vi "Parse CfgTable(with DataName).vi"(7 "Cluster Configuration Typedef":variant, 8 "error in (no error)":errorcluster, 11 "CfgTable Row":string[](array[string])) -> (0 "error out":errorcluster, 1 "Elements":i32, 3 "Cluster Configuration Out":variant)   [LabVIEW 2017, in "ClusterCfgTable.lvlib"]
doc: "NEVSTOP-Programming-Palette 2021.12.23.1\nNEVSTOP - NEVSTOP\nCopyright (c) 2021, NEVSTOP"
uses:
  ClusterCfgTable.lvlib
  <userlib>/_OpenG.lib/string/string.llb/Trim Whitespace (String)__ogtk.vi
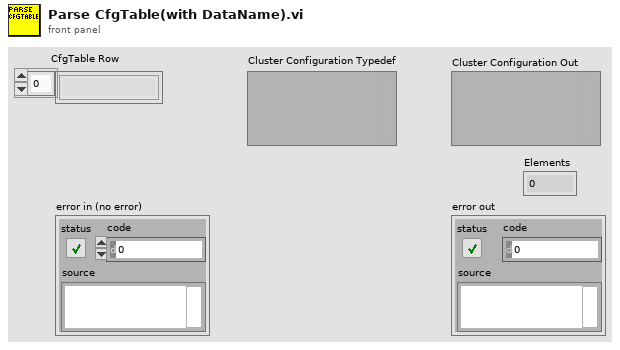
[diagram p1: front panel]
types:
  T1 = typedef "Type Descriptor Enumeration__ogtk.ctl" = enum8{"<Null>", "I8", "I16", "I32", "I64", "U8", "U16", "U32", "U64", "SGL", "DBL", "EXT", "CSG", "CDB", "CXT", "0x0F", "0x10", "0x11", "0x12", "0x13", "0x14", "Enum U8", "Enum U16", "Enum U32", "Enum U64", "SGL PQ", "DBL PQ", "EXT PQ", "CSG PQ", "CDB PQ", "CXT PQ", "0x1F", "0x20", "Boolean", "0x22", "0x23", "0x24", "0x25", "0x26", "0x27", "0x28", "0x29", "0x2A", "0x2B", "0x2C", "0x2D", "0x2E", "0x2F", "String", "0x31", "Path", "Pict", "0x34", "0x35", "0x36", "DAQ", "0x38", "0x39", "0x3A", "0x3B", "0x3C", "0x3D", "0x3E", "0x3F", "Array", "0x41", "0x42", "0x43", "0x44", "0x45", "0x46", "0x47", "0x48", "0x49", "0x4A", "0x4B", "0x4C", "0x4D", "0x4E", "0x4F", "Cluster", "0x51", "0x52", "Variant", "Waveform", "0x55", "0x56", "0x57", "0x58", "0x59", "0x5A", "0x5B", "0x5C", "0x5D", "0x5E", "0x5F", "0x60", "0x61", "0x62", "0x63", "0x64", "0x65", "0x66", "0x67", "0x68", "0x69", "0x6A", "0x6B", "0x6C", "0x6D", "0x6E", "0x6F", "Refnum"}
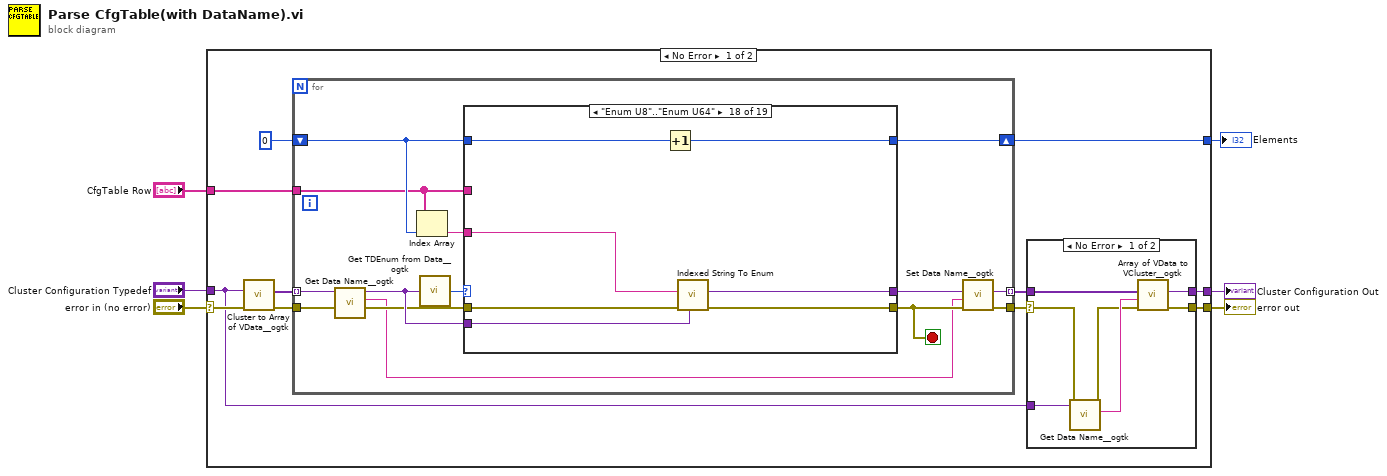
[diagram p0: block diagram]
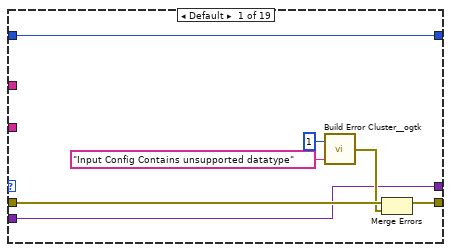
[diagram p3: hidden frame]
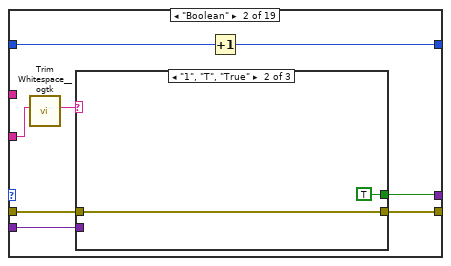
[diagram p4: hidden frame]
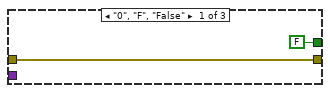
[diagram p5: hidden frame]
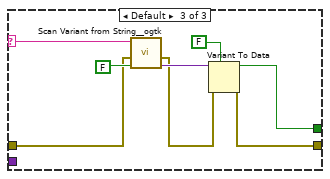
[diagram p6: hidden frame]
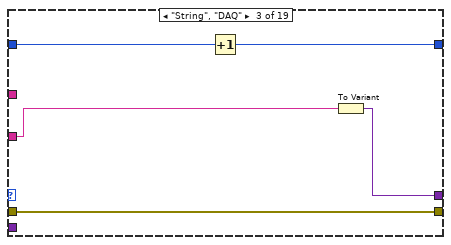
[diagram p7: hidden frame]
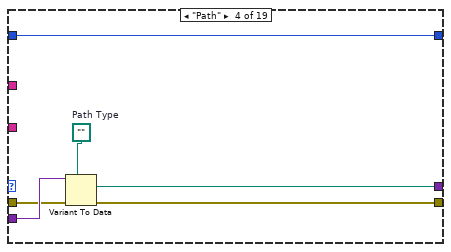
[diagram p8: hidden frame]
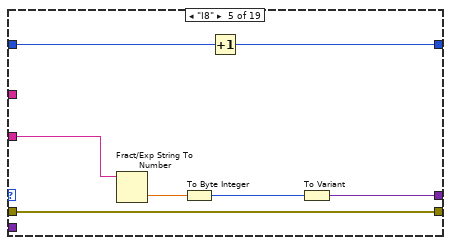
[diagram p9: hidden frame]
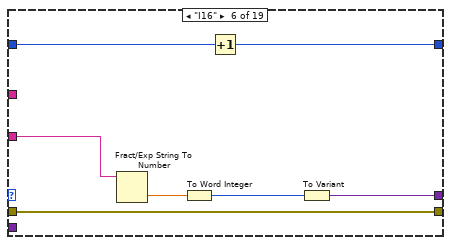
[diagram p10: hidden frame]
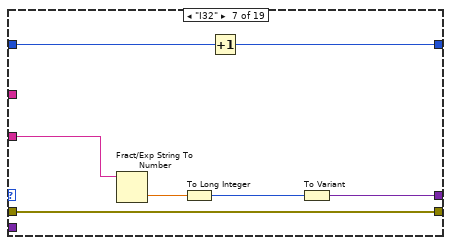
[diagram p11: hidden frame]
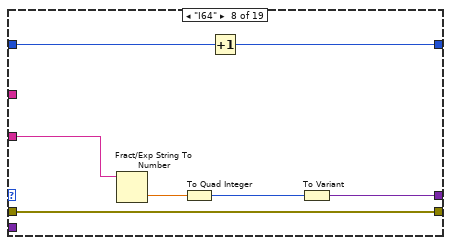
[diagram p12: hidden frame]
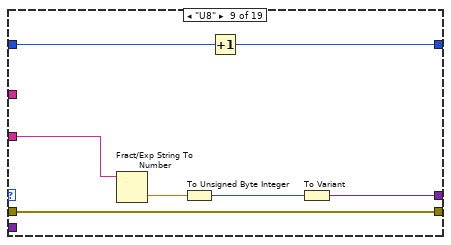
[diagram p13: hidden frame]
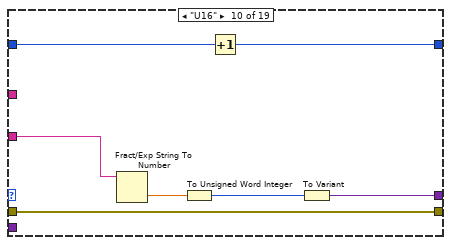
[diagram p14: hidden frame]
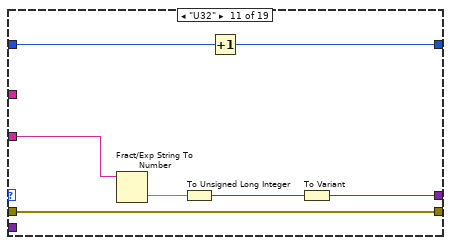
[diagram p15: hidden frame]
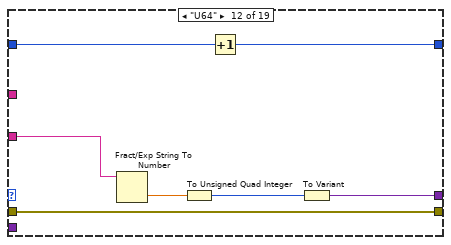
[diagram p16: hidden frame]
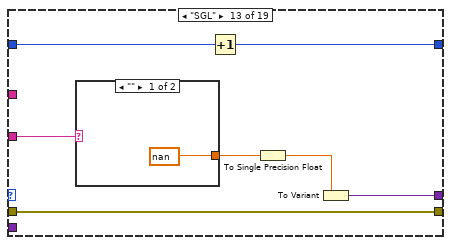
[diagram p17: hidden frame]
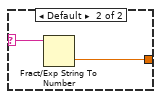
[diagram p18: hidden frame]
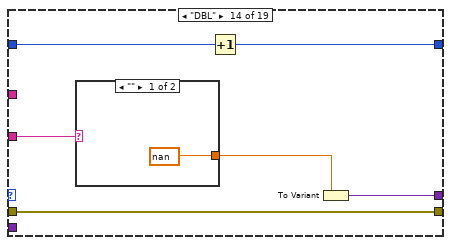
[diagram p19: hidden frame]
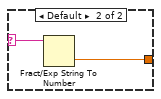
[diagram p20: hidden frame]
diagram:
  n1 = case shown="No Error" "error in (no error)" {
    selector: "error in (no error)" -> [w12 w201]
    tunnel: "CfgTable Row" -> [w17 _]
    tunnel: [w16 w200] -> w5
    tunnel: [w15 w201] -> w4
    tunnel: "Cluster Configuration Typedef" -> [w8 w200]
    tunnel: [w7 _] -> w1
    frame No Error {
      n2 = call <userlib>:"Cluster to Array of VData__ogtk.vi"("error in (no error)"=w12, "Cluster"=w8) -> ("error out"=w13:errorcluster, "Array of VData"=w10:variant[])  [unwired: 8 in]
      n3 = for {
        tunnel: w17 -> [w34]
        tunnel: w10 -> [w37] mode=indexing
        tunnel: [w30] -> w11 mode=indexing
        tunnel: w13 -> [w32]
        tunnel: [w28] -> w14
        shift-right: [w36] -> w7
        shift-left: 0 -> [w35]
        stop <- w29 stop-if-true
        n4 = call <userlib>:"Get Data Name__ogtk.vi"("error in (no error)"=w32, "Data"=w37) -> ("error out"=w31:errorcluster, "Data Name"=w27:string, "Data dup"=w33:variant)  [unwired: 7 in]
        n5 = Index Array(array=w34, index=w35) -> (element=w39:string)
        n6 = call <userlib>:"Get TDEnum from Data__ogtk.vi"("Data"=w33) -> ("Type Descriptor Enumeration"=w40:T1)  [unwired: 4 in]
        n7 = case shown="\"Enum U8\"..\"Enum U64\"" w40 {
          tunnel: w39 -> [_ w55 w72 _ w80 w87 w94 w101 w108 w115 w122 w129 w140 w149 w159 w169 w179 w190 _]
          tunnel: [w42 w53 w71 w74 w85 w92 w99 w106 w113 w120 w127 w134 w141 w150 w160 w170 w180 w189 w195] -> w38
          tunnel: w33 -> [w42 w54 _ w76 _ _ _ _ _ _ _ _ _ _ _ _ _ w188 w196]
          tunnel: w31 -> [w47 w51 w70 w75 w83 w90 w97 w104 w111 w118 w125 w132 w139 w148 w158 w168 w178 w187 w199]
          tunnel: [w46 w50 w70 w73 w83 w90 w97 w104 w111 w118 w125 w132 w139 w148 w158 w168 w178 w186 w192] -> w29
          tunnel: w35 -> [w41 w49 w69 w78 w82 w89 w96 w103 w110 w117 w124 w131 w138 w147 w157 w167 w177 w185 w194]
          tunnel: [w41 w48 w68 w78 w81 w88 w95 w102 w109 w116 w123 w130 w137 w146 w156 w166 w176 w184 w193] -> w36
          tunnel: w34 -> [_ _ _ _ _ _ _ _ _ _ _ _ _ _ _ _ _ _ w198]
          frame Default {
            n8 = call <userlib>:"Build Error Cluster__ogtk.vi"("String to Prepend to source (\"\")"="Input Config Contains unsupported datatype" ("String to Prepend to source (\"\")"), "code"=1) -> ("error out"=w45:errorcluster)
            n9 = Merge Errors(w47, w45) -> (w46:errorcluster)
          }
          frame "Boolean" {
            n10 = call-poly <userlib>:"Trim Whitespace__ogtk.vi"("String in"=w55) -> ("String out"=w52:string)  [unwired: 6 in]
            n11 = case shown="\"1\", \"T\", \"True\"" w52 {
              selector: w52 -> [_ _ w67]
              tunnel: w54 -> [_ _ _]
              tunnel: [FALSE TRUE w64] -> w53
              tunnel: w51 -> [w56 w58 w62]
              tunnel: [w56 w58 w60] -> w50
              frame "0", "F", "False" {
              }
              frame "1", "T", "True" {
              }
              frame Default {
                n12 = call <userlib>:"Scan Variant from String__ogtk.vi"("Default Value"=FALSE, "error in (no error)"=w62, "Input String"=w67) -> ("Output"=w66:variant, "error out"=w61:errorcluster)  [unwired: 5 in, 2 out]
                n13 = Variant To Data(error in=w61, type=FALSE, Variant=w66) -> (data=w64:bool, error out=w60:errorcluster)
              }
            }
            n14 = Increment(x=w49) -> (x+1=w48:i32)
          }
          frame "String", "DAQ" {
            n15 = Increment(x=w69) -> (x+1=w68:i32)
            n16 = To Variant(anything=w72) -> (Variant=w71:variant)
          }
          frame "Path" {
            w77 = path ""  # Path Type
            n17 = Variant To Data(error in=w75, type=w77, Variant=w76) -> (data=w74:path, error out=w73:errorcluster)
          }
          frame "I8" {
            n18 = Fract/Exp String To Number(string=w80) -> (number=w84:dbl)  [unwired: 3 in, 1 out]
            n19 = To Byte Integer(number=w84) -> (8bit integer=w79:i8)
            n20 = Increment(x=w82) -> (x+1=w81:i32)
            n21 = To Variant(anything=w79) -> (Variant=w85:variant)
          }
          frame "I16" {
            n22 = Fract/Exp String To Number(string=w87) -> (number=w91:dbl)  [unwired: 3 in, 1 out]
            n23 = To Word Integer(number=w91) -> (16bit integer=w86:i16)
            n24 = Increment(x=w89) -> (x+1=w88:i32)
            n25 = To Variant(anything=w86) -> (Variant=w92:variant)
          }
          frame "I32" {
            n26 = Fract/Exp String To Number(string=w94) -> (number=w98:dbl)  [unwired: 3 in, 1 out]
            n27 = To Long Integer(number=w98) -> (32bit integer=w93:i32)
            n28 = Increment(x=w96) -> (x+1=w95:i32)
            n29 = To Variant(anything=w93) -> (Variant=w99:variant)
          }
          frame "I64" {
            n30 = Fract/Exp String To Number(string=w101) -> (number=w105:dbl)  [unwired: 3 in, 1 out]
            n31 = To Quad Integer(1:w105) -> (0:w100:i64)
            n32 = Increment(x=w103) -> (x+1=w102:i32)
            n33 = To Variant(anything=w100) -> (Variant=w106:variant)
          }
          frame "U8" {
            n34 = Fract/Exp String To Number(string=w108) -> (number=w112:dbl)  [unwired: 3 in, 1 out]
            n35 = To Unsigned Byte Integer(number=w112) -> (unsigned 8bit integer=w107:u8)
            n36 = Increment(x=w110) -> (x+1=w109:i32)
            n37 = To Variant(anything=w107) -> (Variant=w113:variant)
          }
          frame "U16" {
            n38 = Fract/Exp String To Number(string=w115) -> (number=w119:dbl)  [unwired: 3 in, 1 out]
            n39 = To Unsigned Word Integer(number=w119) -> (unsigned 16bit integer=w114:u16)
            n40 = Increment(x=w117) -> (x+1=w116:i32)
            n41 = To Variant(anything=w114) -> (Variant=w120:variant)
          }
          frame "U32" {
            n42 = Fract/Exp String To Number(string=w122) -> (number=w126:dbl)  [unwired: 3 in, 1 out]
            n43 = To Unsigned Long Integer(number=w126) -> (unsigned 32bit integer=w121:u32)
            n44 = Increment(x=w124) -> (x+1=w123:i32)
            n45 = To Variant(anything=w121) -> (Variant=w127:variant)
          }
          frame "U64" {
            n46 = Fract/Exp String To Number(string=w129) -> (number=w133:dbl)  [unwired: 3 in, 1 out]
            n47 = To Unsigned Quad Integer(1:w133) -> (0:w128:u64)
            n48 = Increment(x=w131) -> (x+1=w130:i32)
            n49 = To Variant(anything=w128) -> (Variant=w134:variant)
          }
          frame "SGL" {
            n50 = case shown="\"\"" w140 {
              selector: w140 -> [_ w144]
              tunnel: [nan ("number") w143] -> w136
              frame "" {
              }
              frame Default {
                n51 = Fract/Exp String To Number(string=w144) -> (number=w143:dbl)  [unwired: 3 in, 1 out]
              }
            }
            n52 = Increment(x=w138) -> (x+1=w137:i32)
            n53 = To Single Precision Float(number=w136) -> (single precision float=w135:sgl)
            n54 = To Variant(anything=w135) -> (Variant=w141:variant)
          }
          frame "DBL" {
            n55 = case shown="\"\"" w149 {
              selector: w149 -> [_ w153]
              tunnel: [nan ("number") w152] -> w145
              frame "" {
              }
              frame Default {
                n56 = Fract/Exp String To Number(string=w153) -> (number=w152:dbl)  [unwired: 3 in, 1 out]
              }
            }
            n57 = Increment(x=w147) -> (x+1=w146:i32)
            n58 = To Variant(anything=w145) -> (Variant=w150:variant)
          }
          frame "SGL PQ" {
            n59 = case shown="Default" w159 {
              selector: w159 -> [_ w163]
              tunnel: [nan ("number") w162] -> w155
              frame "" {
              }
              frame Default {
                n60 = Fract/Exp String To Number(string=w163) -> (number=w162:dbl)  [unwired: 3 in, 1 out]
              }
            }
            n61 = Increment(x=w157) -> (x+1=w156:i32)
            n62 = To Single Precision Complex(1:w155) -> (0:w154:csg)
            n63 = To Variant(anything=w154) -> (Variant=w160:variant)
          }
          frame "DBL PQ" {
            n64 = case shown="Default" w169 {
              selector: w169 -> [_ w173]
              tunnel: [nan ("number") w172] -> w165
              frame "" {
              }
              frame Default {
                n65 = Fract/Exp String To Number(string=w173) -> (number=w172:dbl)  [unwired: 3 in, 1 out]
              }
            }
            n66 = Increment(x=w167) -> (x+1=w166:i32)
            n67 = To Double Precision Complex(1:w165) -> (0:w164:cdb)
            n68 = To Variant(anything=w164) -> (Variant=w170:variant)
          }
          frame "EXT PQ" {
            n69 = case shown="Default" w179 {
              selector: w179 -> [_ w183]
              tunnel: [nan ("number") w182] -> w175
              frame "" {
              }
              frame Default {
                n70 = Fract/Exp String To Number(string=w183) -> (number=w182:dbl)  [unwired: 3 in, 1 out]
              }
            }
            n71 = Increment(x=w177) -> (x+1=w176:i32)
            n72 = To Extended Precision Complex(1:w175) -> (0:w174:cxt)
            n73 = To Variant(anything=w174) -> (Variant=w180:variant)
          }
          frame "Enum U8".."Enum U64" {
            n74 = Increment(x=w185) -> (x+1=w184:i32)
            n75 = call "Indexed String To Enum.vi"("Variant"=w188, "error in (no error)"=w187, "String"=w190) -> ("error out"=w186:errorcluster, "Enum"=w189:variant)  [unwired: 7 in]
          }
          frame "Cluster" {
            n76 = Array Subset(array=w198, index=w194) -> (w197:string[])  [unwired: 1 in]
            n77 = call "Parse CfgTable(with DataName).vi"("Cluster Configuration Typedef"=w196, "error in (no error)"=w199, "CfgTable Row"=w197) -> ("error out"=w192:errorcluster, "Elements"=w191:i32, "Cluster Configuration Out"=w195:variant)  [unwired: 6 in]
            n78 = Add(x=w194, y=w191) -> (x+y=w193:i32)
          }
        }
        n79 = call <userlib>:"Set Data Name__ogtk.vi"("error in (no error)"=w29, "Data Name"=w27, "Data"=w38) -> ("error out"=w28:errorcluster, "Renamed Data"=w30:variant)  [unwired: 7 in]
      }
      n80 = case shown="No Error" w14 {
        selector: w14 -> [w19 w25]
        tunnel: [w24 w26] -> w16
        tunnel: [w23 w25] -> w15
        tunnel: w11 -> [w22 _]
        tunnel: w8 -> [w20 w26]
        frame No Error {
          n81 = call <userlib>:"Get Data Name__ogtk.vi"("error in (no error)"=w19, "Data"=w20) -> ("error out"=w18:errorcluster, "Data Name"=w21:string)  [unwired: 7 in, 1 out]
          n82 = call <userlib>:"Array of VData to VCluster__ogtk.vi"("error in (no error)"=w18, "Cluster Name"=w21, "Array"=w22) -> ("error out"=w23:errorcluster, "VCluster"=w24:variant)  [unwired: 7 in]
        }
        frame Error {
        }
      }
    }
    frame Error {
    }
  }
  "Cluster Configuration Out" <- w5
  "error out" <- w4
  "Elements" <- w1
